vi "atiMatrixMult.vi"(2 "error in (no error)":errorcluster, 3 "Voltages":dbl[](array[numeric]), 4 "Calibration Matrix":dbl[][](array[numeric])) -> (0 "error out":errorcluster, 1 "F/T Data":dbl[](array[numeric]))   [LabVIEW 2019]
doc: "Takes a calibration matrix and voltage vector and mutliplies them to get resolved force/torque data."
uses:
  <vilib>/Analysis/baseanly.llb/A x Vector.vi
  <vilib>/Analysis/NI_AALBase.lvlib
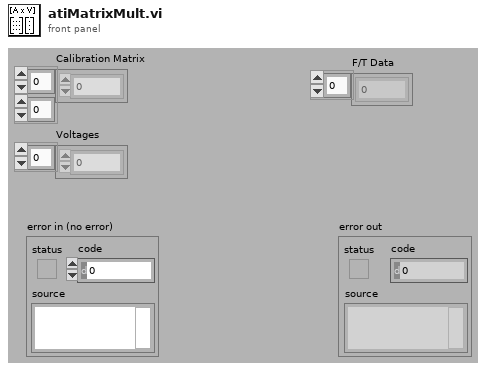
[diagram p1: front panel]
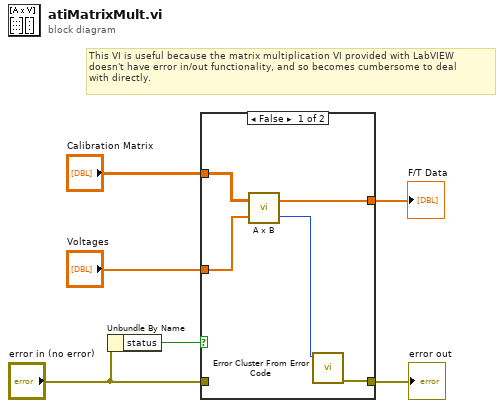
[diagram p0: block diagram]
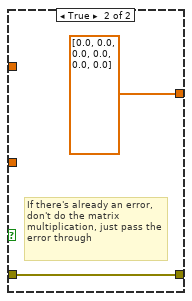
[diagram p2: hidden frame]
diagram:
  # "This VI is useful because the matrix multiplication VI provided with LabVIEW\ndoesn't have error in/out functionality, and so becomes cumbersome to deal\nwith directly."
  n1 = Unbundle By Name("error in (no error)") -> ("status"=w4:bool)
  n2 = case shown="False" w4 {
    tunnel: [w8 w13] -> w6
    tunnel: "error in (no error)" -> [_ w13]
    tunnel: "Calibration Matrix" -> [w11 _]
    tunnel: "Voltages" -> [w10 _]
    tunnel: [w7 dbl[] [0.0, 0.0, 0.0, 0.0, 0.0, 0.0]] -> w1
    frame False {
      n3 = call-poly <vilib>:"A x B.vi"("Vector"=w10, "A"=w11) -> ("error"=w9:i32, "A x Vector"=w7:dbl[])
      n4 = call <vilib>:"Error Cluster From Error Code.vi"("error code (0)"=w9) -> ("error out"=w8:errorcluster)  [unwired: 8 in]
    }
    frame True {
      # "If there's already an error, \ndon't do the matrix\nmultiplication, just pass the\nerror through"
    }
  }
  "error out" <- w6
  "F/T Data" <- w1
